vi "GetRelEncPos.vi"(11 "Update?":bool) -> (0 "RearRightQuadPos":i32, 1 "RearLeftQuadPos":i32, 2 "FrontRightQuadPos":i32, 3 "FrontLeftQuadPos":i32, 8 "error in":errorcluster)   [LabVIEW 2018]
uses:
  <vilib>/Rock Robotics/WPI/ThirdParty/Phoenix-LabVIEW/Motor Controller/Get/CTRE_Phoenix_MotorController_GetQuadratureData.vi
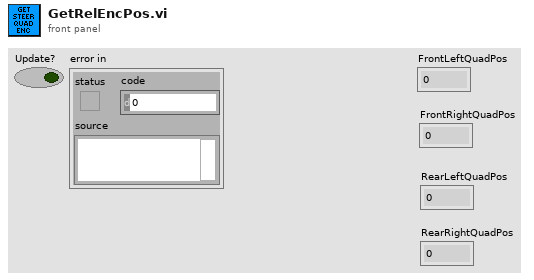
[diagram p1: front panel]
types:
  T1 = typedef "WPI_MotorControlDeviceRef.ctl" = cluster{"DeviceStatus":errorcluster, "Type":T2, "PWM":cluster{"PWM Channel":T3, "DeadBand":T4}, "CAN":cluster{"Device Number":u8, "SetOutput VI Ref":variant, "GetOutput VI Ref":variant, "Enable VI Ref":variant, "Disable VI Ref":variant, "Data":variant}, "Invert":bool, "DIO PWM":cluster{"PWM \"Enable\" Channel":T3, "DIOChannel":T5, "PWM Rate":dbl}}
  T2 = typedef "WPI_MotorControlType.ctl" = enum16{"PWM", "CAN", "DIO PWM"}
  T3 = typedef "FPGA_DIOPWMChannel.ctl" = enum8{"PWM 0", "PWM 1", "PWM 2", "PWM 3", "PWM 4", "PWM 5", "PWM 6", "PWM 7", "PWM 8", "PWM 9", "PWM MXP 0", "PWM MXP 1", "PWM MXP 2", "PWM MXP 3", "PWM MXP 4", "PWM MXP 5", "PWM MXP 6", "PWM MXP 7", "PWM MXP 8", "PWM MXP 9", "Invalid"}
  T4 = typedef "WPI_PWMDeadband.ctl" = cluster{"Name":string, "maxPositivePwm":i32, "minPositivePwm":i32, "centerPwm":i32, "maxNegativePwm":i32, "minNegativePwm":i32, "angularRange":u16}
  T5 = typedef "FPGA_DIOChannel.ctl" = enum8{"DIO 0", "DIO 1", "DIO 2", "DIO 3", "DIO 4", "DIO 5", "DIO 6", "DIO 7", "DIO 8", "DIO 9", "DIO MXP 0", "DIO MXP 1", "DIO MXP 2", "DIO MXP 3", "DIO MXP 4", "DIO MXP 5", "DIO MXP 6", "DIO MXP 7", "DIO MXP 8", "DIO MXP 9", "DIO MXP 10", "DIO MXP 11", "DIO MXP 12", "DIO MXP 13", "DIO MXP 14", "DIO MXP 15", "SPI Port CS1", "SPI Port CS2", "SPI Port CS3", "SPI Port MISO", "SPI Port MOSI", "Invalid"}
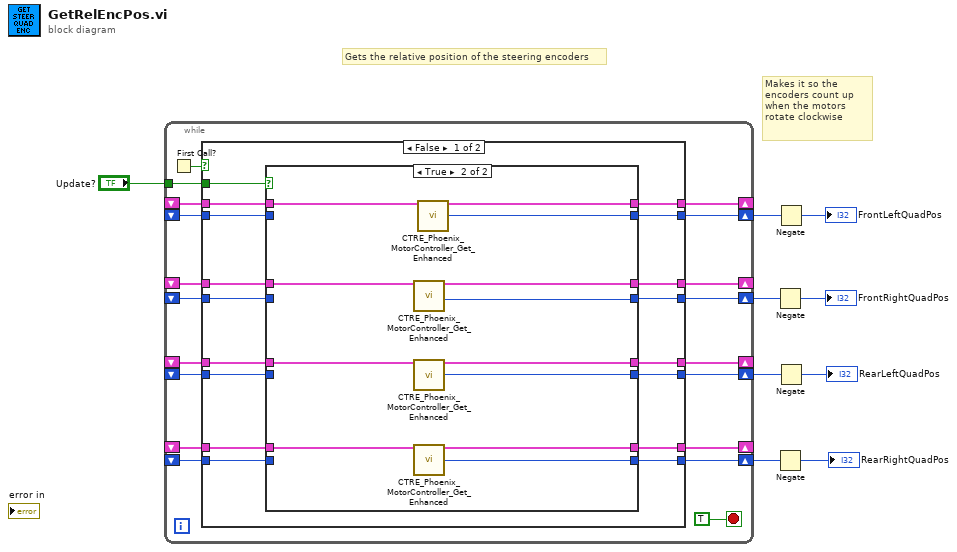
[diagram p0: block diagram]
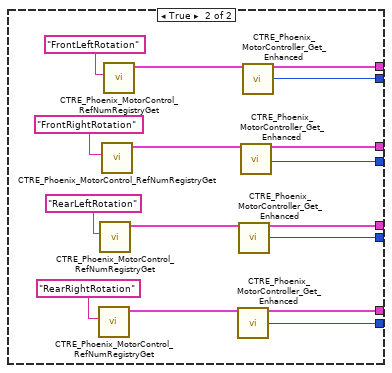
[diagram p3: hidden frame]
diagram:
  # "Gets the relative position of the steering encoders"
  # "Makes it so the encoders count up when the motors rotate clockwise"
  n1 = while {
    shift-right: [w27] -> _
    shift-left: _ -> [w26]
    tunnel: "Update?" -> [w24]
    shift-right: [w28] -> w7
    shift-left: _ -> [w23]
    shift-right: [w22] -> _
    shift-left: _ -> [w16]
    shift-right: [w21] -> w1
    shift-left: _ -> [w13]
    shift-right: [w20] -> _
    shift-left: _ -> [w15]
    shift-right: [w19] -> w3
    shift-left: _ -> [w12]
    shift-right: [w18] -> _
    shift-left: _ -> [w14]
    shift-right: [w17] -> w5
    shift-left: _ -> [w11]
    stop <- TRUE stop-if-true
    n2 = First Call?() -> (First Call?: T/F=w25:bool)
    n3 = case shown="False" w25 {
      tunnel: w26 -> [w45 _]
      tunnel: [w44 w78] -> w28
      tunnel: [w43 w79] -> w27
      tunnel: w24 -> [w42 _]
      tunnel: w23 -> [w41 _]
      tunnel: [w39 w71] -> w22
      tunnel: [w34 w70] -> w21
      tunnel: [w38 w69] -> w20
      tunnel: [w33 w68] -> w19
      tunnel: [w35 w67] -> w18
      tunnel: [w32 w66] -> w17
      tunnel: w16 -> [w40 _]
      tunnel: w15 -> [w37 _]
      tunnel: w14 -> [w36 _]
      tunnel: w13 -> [w31 _]
      tunnel: w12 -> [w30 _]
      tunnel: w11 -> [w29 _]
      frame False {
        n4 = case shown="True" w42 {
          tunnel: w45 -> [w53 w65]
          tunnel: [w52 w64] -> w44
          tunnel: [w53 w63] -> w43
          tunnel: w41 -> [w52 _]
          tunnel: w40 -> [w51 w62]
          tunnel: [w51 w61] -> w39
          tunnel: [w50 w60] -> w38
          tunnel: w37 -> [w50 w59]
          tunnel: w36 -> [w49 w58]
          tunnel: [w49 w57] -> w35
          tunnel: [w48 w56] -> w34
          tunnel: [w47 w55] -> w33
          tunnel: [w46 w54] -> w32
          tunnel: w31 -> [w48 _]
          tunnel: w30 -> [w47 _]
          tunnel: w29 -> [w46 _]
          frame False {
          }
          frame True {
            n5 = call-poly <vilib>:"CTRE_Phoenix_MotorController_Get_Enhanced.vi"("PhoenixMotorControlDevRef"=w62) -> ("PhoenixMotorControlDevRef"=w61:T1, "Quadrature Position"=w56:i32)  [unwired: 11 in, 2 out]
            n6 = call-poly <vilib>:"CTRE_Phoenix_MotorController_Get_Enhanced.vi"("PhoenixMotorControlDevRef"=w59) -> ("PhoenixMotorControlDevRef"=w60:T1, "Quadrature Position"=w55:i32)  [unwired: 11 in, 2 out]
            n7 = call-poly <vilib>:"CTRE_Phoenix_MotorController_Get_Enhanced.vi"("PhoenixMotorControlDevRef"=w58) -> ("PhoenixMotorControlDevRef"=w57:T1, "Quadrature Position"=w54:i32)  [unwired: 11 in, 2 out]
            n8 = call-poly <vilib>:"CTRE_Phoenix_MotorController_Get_Enhanced.vi"("PhoenixMotorControlDevRef"=w65) -> ("PhoenixMotorControlDevRef"=w63:T1, "Quadrature Position"=w64:i32)  [unwired: 11 in, 2 out]
          }
        }
      }
      frame True {
        n9 = call <vilib>:"CTRE_Phoenix_MotorControl_RefNumRegistryGet.vi"("refnum name"="RearRightRotation") -> ("PhoenixMotorControlDevRef"=w73:T1)  [unwired: 9 in, 1 out]
        n10 = call <vilib>:"CTRE_Phoenix_MotorControl_RefNumRegistryGet.vi"("refnum name"="RearLeftRotation") -> ("PhoenixMotorControlDevRef"=w74:T1)  [unwired: 9 in, 1 out]
        n11 = call <vilib>:"CTRE_Phoenix_MotorControl_RefNumRegistryGet.vi"("refnum name"="FrontRightRotation") -> ("PhoenixMotorControlDevRef"=w77:T1)  [unwired: 9 in, 1 out]
        n12 = call <vilib>:"CTRE_Phoenix_MotorControl_RefNumRegistryGet.vi"("refnum name"="FrontLeftRotation") -> ("PhoenixMotorControlDevRef"=w80:T1)  [unwired: 9 in, 1 out]
        n13 = call-poly <vilib>:"CTRE_Phoenix_MotorController_Get_Enhanced.vi"("PhoenixMotorControlDevRef"=w73) -> ("PhoenixMotorControlDevRef"=w67:T1, "Quadrature Position"=w66:i32)  [unwired: 11 in, 2 out]
        n14 = call-poly <vilib>:"CTRE_Phoenix_MotorController_Get_Enhanced.vi"("PhoenixMotorControlDevRef"=w74) -> ("PhoenixMotorControlDevRef"=w69:T1, "Quadrature Position"=w68:i32)  [unwired: 11 in, 2 out]
        n15 = call-poly <vilib>:"CTRE_Phoenix_MotorController_Get_Enhanced.vi"("PhoenixMotorControlDevRef"=w77) -> ("PhoenixMotorControlDevRef"=w71:T1, "Quadrature Position"=w70:i32)  [unwired: 11 in, 2 out]
        n16 = call-poly <vilib>:"CTRE_Phoenix_MotorController_Get_Enhanced.vi"("PhoenixMotorControlDevRef"=w80) -> ("PhoenixMotorControlDevRef"=w79:T1, "Quadrature Position"=w78:i32)  [unwired: 11 in, 2 out]
      }
    }
  }
  n17 = Negate(x=w1) -> (-x=→"FrontRightQuadPos":i32)
  n18 = Negate(x=w5) -> (-x=→"RearRightQuadPos":i32)
  n19 = Negate(x=w7) -> (-x=→"FrontLeftQuadPos":i32)
  n20 = Negate(x=w3) -> (-x=→"RearLeftQuadPos":i32)
